vi "Runtime Test.vi"() -> (0 "final error":errorcluster, 1 "correct execution settings":bool, 2 "Pass Input":bool[](array[boolean]), 3 "Pass Output":bool[](array[boolean]))   [LabVIEW 2015, in "SystemLink Tag Module tests.lvlib"]
doc: "This VI shows an example for how to test the Runtime functionality of the module. This will need to be modified according to module functionality."
uses:
  SystemLink Tag Module tests.lvlib
  module/execution/SystemLink runtime.lvclass
  module/configuration/SystemLink configuration.lvclass
panel:
  out "Names":string[](array[string])
  out "init error":errorcluster
  out "invalid configuration":errorcluster
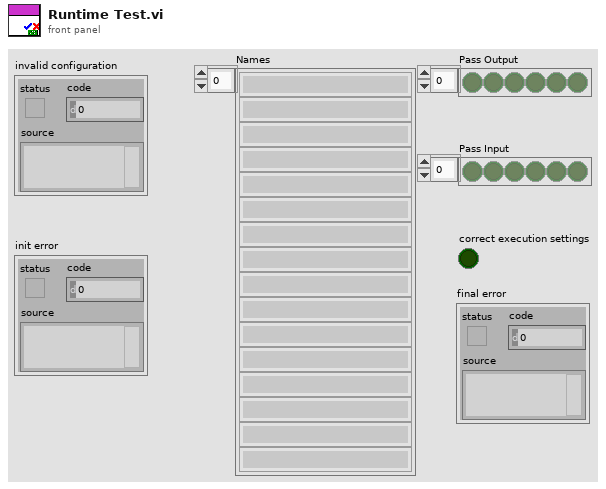
[diagram p1: front panel]
types:
  T1 = typedef "TBM channel.lvclass/data tables.ctl" = cluster{"input data":T2, "processing parameter":T2, "processing result":T2, "output data":T2}
  T2 = typedef "tag bus.lvlib/dictionary table pair.ctl" = cluster{"data dictionary":refnum<class "data dictionary.lvclass">, "data table":T3}
  T3 = typedef "tag bus.lvlib/data table.lvlib/data table.ctl" = cluster{"Double":dbl[], "Single":sgl[], "I64":i64[], "I32":i32[], "I16":i16[], "I8":i8[], "U64":u64[], "U32":u32[], "U16":u16[], "U8":u8[], "Boolean":bool[], "String":string[], "Array of Double":cluster{"DBL Array":dbl[]}[], "Array of Single":cluster{"SGL Array":sgl[]}[], "Array of I64":cluster{"I64 Array":i64[]}[], "Array of I32":cluster{"I32 Array":i32[]}[], "Array of I16":cluster{"I16 Array":i16[]}[], "Array of I8":cluster{"I8 Array":i8[]}[], "Array of U64":cluster{"U64 Array":u64[]}[], "Array of U32":cluster{"U32 Array":u32[]}[], "Array of U16":cluster{"U16 Array":u16[]}[], "Array of U8":cluster{"U8 Array":u8[]}[], "Array of Boolean":cluster{"Boolean Array":bool[]}[], "Array of String":cluster{"String Array":string[]}[]}
  T4 = typedef "TBM module execution interface.lvclass/execution settings.ctl" = cluster{"reads inputs":bool, "processes data":bool, "writes outputs":bool}
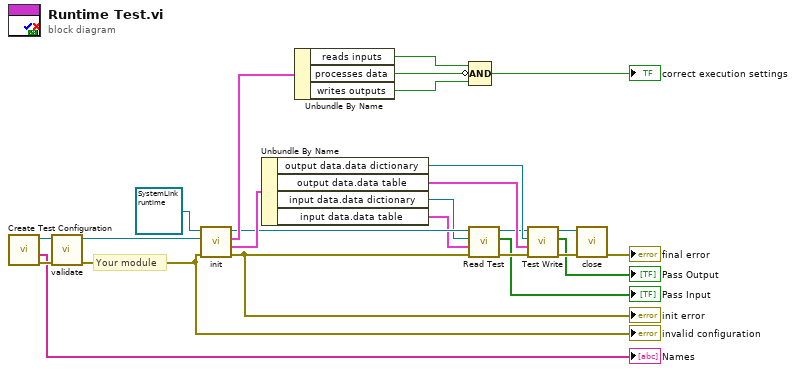
[diagram p0: block diagram]
diagram:
  # "Your module"
  n1 = call "Create Test Configuration.vi"() -> ("error out"=w6:errorcluster, "Names"=→"Names":string[], "Module Configuration"=w7:refnum<class "SystemLink configuration.lvclass">)  [unwired: 6 in, 3 out]
  n2 = call-dynamic "validate.vi"("error in"=w6, "SystemLin Tag Module configuration in"=w7) -> ("error out"=w24:errorcluster, "SystemLin Tag Module configuration out"=w25:refnum<class "SystemLink configuration.lvclass">)  [unwired: 8 in]
  "invalid configuration" <- w24
  n3 = call-dynamic "init.vi"("error in"=w24, "TBM module configuration in"=w25, "SystemLin Tag Module runtime in"=refnum<class "SystemLink runtime.lvclass"> refnum ("tag bus configurable plugin module")) -> ("error out"=w16:errorcluster, "data allocations"=w17:T1, "execution settings"=w22:T4, "SystemLin Tag Module runtime out"=w15:refnum<class "SystemLink runtime.lvclass">)  [unwired: 5 in]
  "init error" <- w16
  n4 = Unbundle By Name(w17) -> ("output data.data dictionary"=w14:refnum<class "data dictionary.lvclass">, "output data.data table"=w13:T3, "input data.data dictionary"=w1:refnum<class "data dictionary.lvclass">, "input data.data table"=w2:T3)
  n5 = Unbundle By Name(w22) -> ("reads inputs"=w19:bool, "processes data"=w21:bool, "writes outputs"=w20:bool)
  n6 = Compound Arithmetic op=AND(w19, invert w21, w20) -> (→"correct execution settings":bool)
  n7 = call "Read Test.vi"("error in (no error)"=w16, "data table"=w2, "data dictionary"=w1, "runtime in"=w15) -> ("error out"=w12:errorcluster, "Pass"=→"Pass Input":bool[], "runtime out"=w11:refnum<class "SystemLink runtime.lvclass">)  [unwired: 5 in]
  n8 = call "Test Write.vi"("error in (no error)"=w12, "data table"=w13, "data dictionary"=w14, "runtime in"=w11) -> ("error out"=w9:errorcluster, "Pass"=→"Pass Output":bool[], "runtime out"=w10:refnum<class "SystemLink runtime.lvclass">)  [unwired: 4 in, 1 out]
  n9 = call-dynamic "close.vi"("error in"=w9, "SystemLin Tag Module runtime in"=w10) -> ("error out"=→"final error":errorcluster)  [unwired: 9 in]
